vi "SensingTransform_v5.vi"(8 "1/Sensing Radius":fxp<+,18,0>, 9 "Pos3 (Left, B)":fxp<+/-,25,3>, 10 "Pos2 (Right, G)":fxp<+/-,25,3>, 11 "Pos1 (Top, R)":fxp<+/-,25,3>) -> (1 "Theta Y [rad]":fxp<+/-,26,3> format="%.8f", 2 "Theta X [rad]":fxp<+/-,26,3> format="%.8f", 3 "Z position":fxp<+/-,26,3> format="%.8f")   [LabVIEW 2020, in "FPGA functions.lvlib"]
doc: "Sensing transformation block\n\nFor 3 sensors placed radially symmetrically, translates into average distance (air-gap) and angles along the plane.\n\nv3: Reduced number of multiplication blocks required, used SCTL"
uses:
  FPGA functions.lvlib
  <vilib>/Platform/TimedLoop/XDataNode/timing_clust.ctl
  <vilib>/Platform/TimedLoop/XDataNode/nitl_modes.ctl
  <vilib>/Platform/TimedLoop/XDataNode/wakeup.ctl
  <vilib>/rvi/Emulation/niFpgaSctlEmulationGetInTimedLoop.vi
  <vilib>/rvi/Emulation/niFpgaEmulationReportErrorSimple.vi
  <vilib>/rvi/Emulation/niFpgaGetClockAttributes.vi
  <vilib>/rvi/Emulation/niFpgaCriticalErrorInLSC.vi
  <vilib>/Platform/TimedLoop/XDataNode/XDataNode.xnode
  <vilib>/rvi/FXPMathLib/FxpSub/XNode/nifxpmath_Sub.xnode
  <vilib>/rvi/FXPMathLib/FxpMul/XNode/nifxpmath_Multiplier.xnode
  <vilib>/rvi/FXPMathLib/FxpAdd/XNode/nifxpmath_Add.xnode
  <vilib>/rvi/FXPMathLib/sim/FxpSim.dll
  <vilib>/Platform/TimedLoop/XDataNode/XDNodeRunTimeDep.lvlib
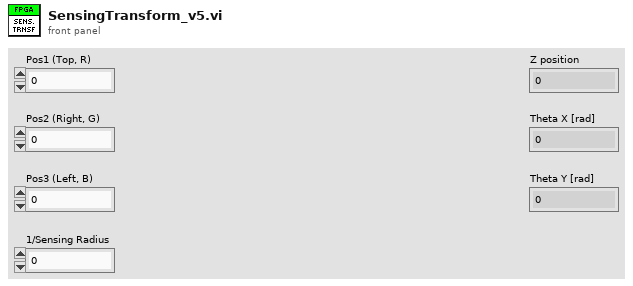
[diagram p1: front panel]
types:
  T1 = typedef "XDNodeRunTimeDep.lvlib/timing_clust.ctl" = cluster{"Expected End [f-1]":u64, "Actual End [f-1]":u64, "Finished Late? [f-1]":bool, "Expected End [i-1]":u64, "Actual End [i-1]":u64, "Finished Late? [i-1]":bool, "Expected Start [i]":u64, "Actual Start [i]":u64, "Expected Start [f]":u64, "Actual Start [f]":u64, "Source Name":string, "Structure Name":string, "Period":i64, "Deadline":i64, "Offset":i64, "Start":i64, "Priority":i32, "Timeout":i32, "Mode":T2, "Wakeup Reason":T3, "Error":errorcluster, "Source Type":string, "Secondary Source Type":string, "Global End Time":u64, "Global Start Time":u64, "Frame Duration":u64, "Iteration Duration":u64, "Assigned CPU":i32, "I/O Scan Engine Mode":u32}
  T2 = typedef "XDNodeRunTimeDep.lvlib/nitl_modes.ctl" = enum32{"No Change", "Process missed periods, maintain original phase", "Discard missed periods, maintain original phase", "Process missed periods, ignore original phase", "Discard missed periods, ignore original phase"}
  T3 = typedef "XDNodeRunTimeDep.lvlib/wakeup.ctl" = enum32{"Normal", "Aborted", "Asynchronous wakeup", "Timing source error", "Timed loop error", "Timeout"}
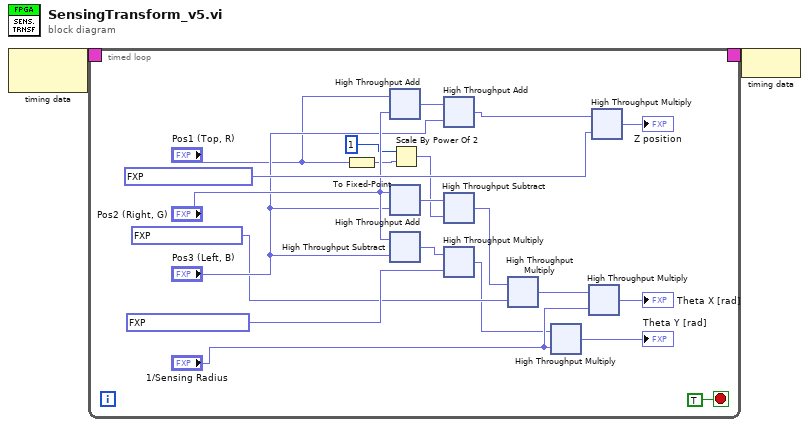
[diagram p0: block diagram]
diagram:
  n1 = node-c288() -> (w2:T1)  [unwired: 1 in]
  n2 = timed-loop {
    timing: w2 -> [_]
    timing-out: [_] -> w1
    stop <- TRUE stop-if-true
    n3 = To Fixed-Point(number="Pos1 (Top, R)") -> (fixed-point=w6:fxp<+/-,26,4>)  [unwired: 1 in]
    n4 = xnode ("High Throughput Add")("x"="Pos1 (Top, R)", "y"="Pos2 (Right, G)") -> ("x+y"=w13:fxp<+/-,26,4>)
    n5 = xnode ("High Throughput Add")("x"="Pos2 (Right, G)", "y"="Pos3 (Left, B)") -> ("x+y"=w8:fxp<+/-,26,4>)
    n6 = xnode ("High Throughput Subtract")("x"="Pos2 (Right, G)", "y"="Pos3 (Left, B)") -> ("x-y"=w14:fxp<+/-,25,4>)
    n7 = Scale By Power Of 2(n=i16 1, x=w6) -> (x*2^n=w7:fxp<+/-,26,4>)
    n8 = xnode ("High Throughput Add")("x"=w13, "y"="Pos3 (Left, B)") -> ("x+y"=w9:fxp<+/-,25,5>)
    n9 = xnode ("High Throughput Subtract")("x"=w8, "y"=w7) -> ("x-y"=w12:fxp<+/-,25,5>)
    n10 = xnode ("High Throughput Multiply")("x"=w14, "y"=fxp<+,18,0> 0.5773506164550781) -> ("x*y"=w10:fxp<+/-,27,4>)
    n11 = xnode ("High Throughput Multiply")("x"=w12, "y"=fxp<+,18,0> 0.3333282470703125) -> ("x*y"=w11:fxp<+/-,27,4>)
    n12 = xnode ("High Throughput Multiply")("x"=w10, "y"="1/Sensing Radius") -> ("x*y"=→"Theta Y [rad]":fxp<+/-,26,3>)
    n13 = xnode ("High Throughput Multiply")("x"=w11, "y"="1/Sensing Radius") -> ("x*y"=→"Theta X [rad]":fxp<+/-,26,3>)
    n14 = xnode ("High Throughput Multiply")("x"=w9, "y"=fxp<+/-,18,0> -0.3333320617675781) -> ("x*y"=→"Z position":fxp<+/-,26,3>)
  }
  n15 = node-c288(w1) -> ()
